vi "Limit Switches.vi"(1 "Backward Limit Switch":bool, 2 "VBus in":dbl, 3 "Forward Limit Switch":bool) -> (0 "VBus out":dbl)   [LabVIEW 2012]
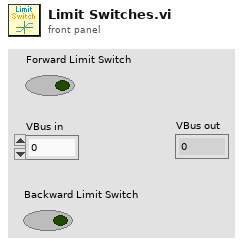
[diagram p1: front panel]
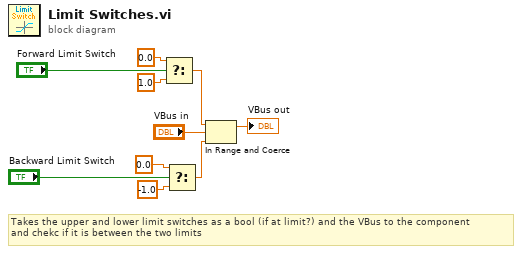
[diagram p0: block diagram]
diagram:
  # "Takes the upper and lower limit switches as a bool (if at limit?) and the VBus to the component \nand chekc if it is between the two limits"
  n1 = Select(t=0.0, s="Forward Limit Switch", f=1.0) -> (s? t:f=w9:dbl)
  n2 = Select(t=0.0, s="Backward Limit Switch", f=-1.0) -> (s? t:f=w8:dbl)
  n3 = In Range and Coerce(upper limit=w9, x="VBus in", lower limit=w8) -> (coerced(x)=→"VBus out":dbl)  [unwired: 1 out]
